vi "keccak.fpga.step.10-14.vi"(6 "Step.8.Dx":u64[](array[numeric])=[0, 0, 0, 0, 0], 9 "Exy.in":u64[](array[numeric])=[0, 0, 0, 0, 0, 0, 0, 0, 0, 0, 0, 0, 0, 0, 0, 0, 0, 0, 0, 0, 0, 0, 0, 0, 0] format="%.0x", 10 "D.Indexes":i32[](array[numeric])=[0, 0, 0, 0, 0], 11 "Left Shifts":i32[](array[numeric])=[0, 0, 0, 0, 0]) -> (3 "New.State":u64[](array[numeric]) format="%.0x")   [LabVIEW 2021]
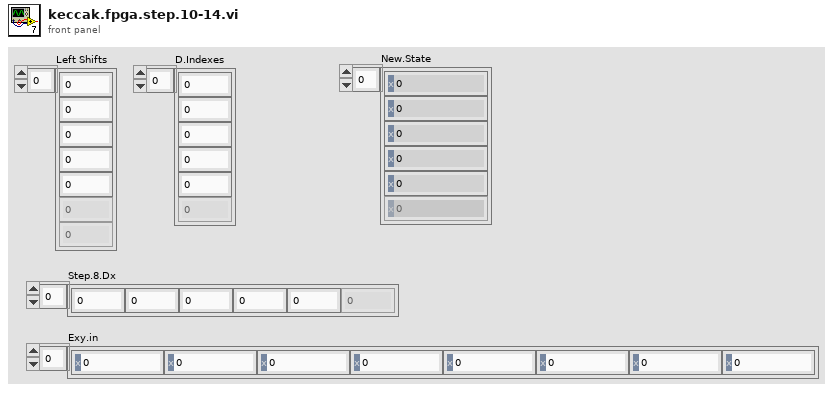
[diagram p1: front panel]
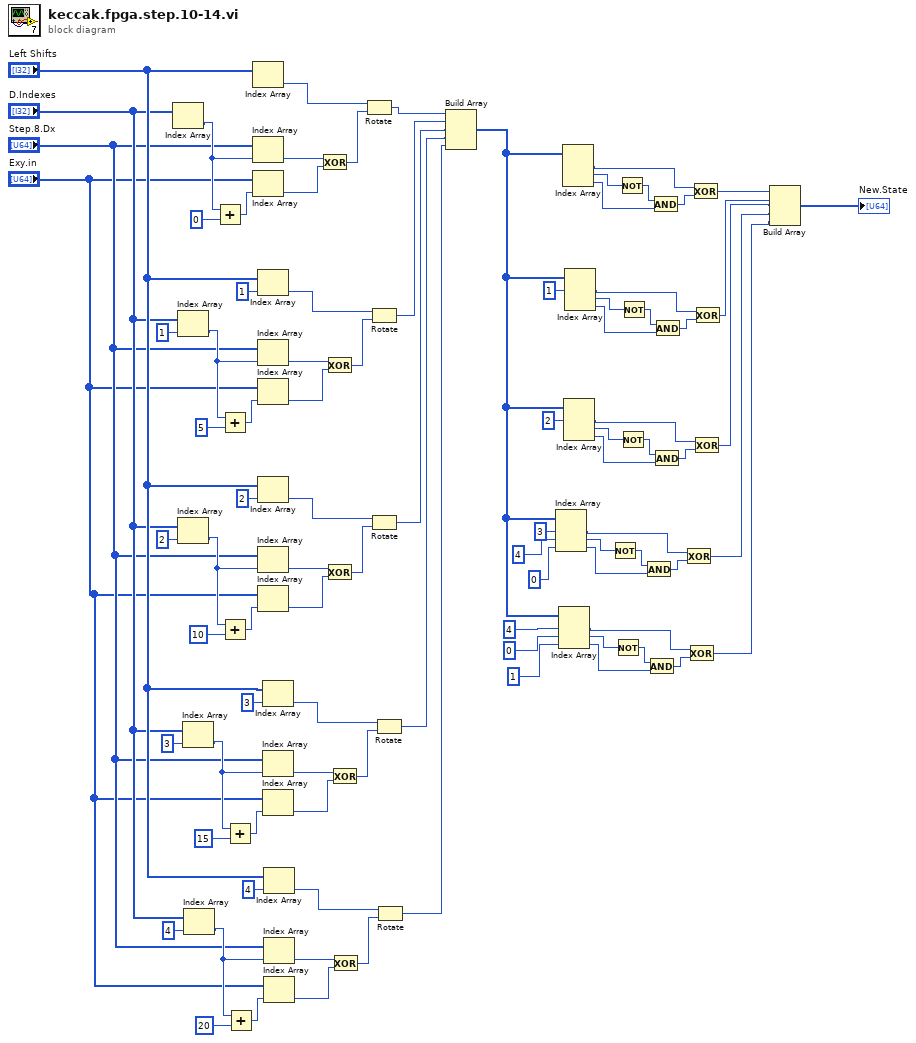
[diagram p0: block diagram]
diagram:
  n1 = Index Array(array="D.Indexes") -> (element=w87:i32)  [unwired: 1 in]
  n2 = Index Array(array="D.Indexes", index=1) -> (element=w72:i32)
  n3 = Index Array(array="D.Indexes", index=2) -> (element=w62:i32)
  n4 = Index Array(array="D.Indexes", index=3) -> (element=w52:i32)
  n5 = Index Array(array="D.Indexes", index=4) -> (element=w43:i32)
  n6 = Add(x=w87, y=0 ("x")) -> (x+y=w92:i32)
  n7 = Add(x=w72, y=5 ("x")) -> (x+y=w77:i32)
  n8 = Add(x=w62, y=10 ("x")) -> (x+y=w67:i32)
  n9 = Add(x=w52, y=15 ("x")) -> (x+y=w57:i32)
  n10 = Add(x=w43, y=20 ("x")) -> (x+y=w48:i32)
  n11 = Index Array(array="Left Shifts") -> (element=w88:i32)  [unwired: 1 in]
  n12 = Index Array(array="Step.8.Dx", index=w87) -> (element=w90:u64)
  n13 = Index Array(array="Exy.in", index=w92) -> (element=w91:u64)
  n14 = Index Array(array="Left Shifts", index=1) -> (element=w73:i32)
  n15 = Index Array(array="Step.8.Dx", index=w72) -> (element=w75:u64)
  n16 = Index Array(array="Exy.in", index=w77) -> (element=w76:u64)
  n17 = Index Array(array="Left Shifts", index=2) -> (element=w63:i32)
  n18 = Index Array(array="Step.8.Dx", index=w62) -> (element=w65:u64)
  n19 = Index Array(array="Exy.in", index=w67) -> (element=w66:u64)
  n20 = Index Array(array="Left Shifts", index=3) -> (element=w53:i32)
  n21 = Index Array(array="Step.8.Dx", index=w52) -> (element=w55:u64)
  n22 = Index Array(array="Exy.in", index=w57) -> (element=w56:u64)
  n23 = Index Array(array="Left Shifts", index=4) -> (element=w44:i32)
  n24 = Index Array(array="Step.8.Dx", index=w43) -> (element=w46:u64)
  n25 = Index Array(array="Exy.in", index=w48) -> (element=w47:u64)
  n26 = Exclusive Or(1:w91, 2:w90) -> (0:w89:u64)
  n27 = Exclusive Or(1:w76, 2:w75) -> (0:w74:u64)
  n28 = Exclusive Or(1:w66, 2:w65) -> (0:w64:u64)
  n29 = Exclusive Or(1:w56, 2:w55) -> (0:w54:u64)
  n30 = Exclusive Or(1:w47, 2:w46) -> (0:w45:u64)
  n31 = Rotate(1:w89, 2:w88) -> (0:w85:u64)
  n32 = Rotate(1:w74, 2:w73) -> (0:w68:u64)
  n33 = Rotate(1:w64, 2:w63) -> (0:w58:u64)
  n34 = Rotate(1:w54, 2:w53) -> (0:w39:u64)
  n35 = Rotate(1:w45, 2:w44) -> (0:w38:u64)
  n36 = Build Array(w85, w68, w58, w39, w38) -> (w13:u64[])
  n37 = Index Array(array=w13, index #1=3 ("index"), index #2=4 ("index"), index #3=0 ("index")) -> (element #1=w20:u64, element #2=w23:u64, element #3=w21:u64)
  n38 = Index Array(array=w13, index #1=4 ("index"), index #2=0 ("index"), index #3=1 ("index")) -> (element #1=w15:u64, element #2=w18:u64, element #3=w16:u64)
  n39 = Index Array(array=w13) -> (element #1=w81:u64, element #2=w84:u64, element #3=w82:u64)  [unwired: 3 in]
  n40 = Index Array(array=w13, index #1=2 ("index")) -> (element #1=w25:u64, element #2=w28:u64, element #3=w26:u64)  [unwired: 2 in]
  n41 = Index Array(array=w13, index #1=1 ("index")) -> (element #1=w30:u64, element #2=w33:u64, element #3=w31:u64)  [unwired: 2 in]
  n42 = Not(x=w23) -> (.not. x?=w22:u64)
  n43 = Not(x=w18) -> (.not. x?=w17:u64)
  n44 = Not(x=w84) -> (.not. x?=w83:u64)
  n45 = Not(x=w28) -> (.not. x?=w27:u64)
  n46 = Not(x=w33) -> (.not. x?=w32:u64)
  n47 = And(x=w22, y=w21) -> (x .and. y?=w19:u64)
  n48 = And(x=w17, y=w16) -> (x .and. y?=w14:u64)
  n49 = And(x=w83, y=w82) -> (x .and. y?=w80:u64)
  n50 = And(x=w27, y=w26) -> (x .and. y?=w24:u64)
  n51 = And(x=w32, y=w31) -> (x .and. y?=w29:u64)
  n52 = Exclusive Or(1:w19, 2:w20) -> (0:w10:u64)
  n53 = Exclusive Or(1:w14, 2:w15) -> (0:w9:u64)
  n54 = Exclusive Or(1:w80, 2:w81) -> (0:w79:u64)
  n55 = Exclusive Or(1:w24, 2:w25) -> (0:w11:u64)
  n56 = Exclusive Or(1:w29, 2:w30) -> (0:w12:u64)
  n57 = Build Array(w79, w12, w11, w10, w9) -> (→"New.State":u64[])
